vi "Is it a hex string.vi"(8 "error in (no error)":errorcluster, 9 "length (rest)":i32, 10 "String offset":u32, 11 "String to check":string) -> (0 "error out":errorcluster, 3 "Is Hex string?":bool)   [LabVIEW 2013]
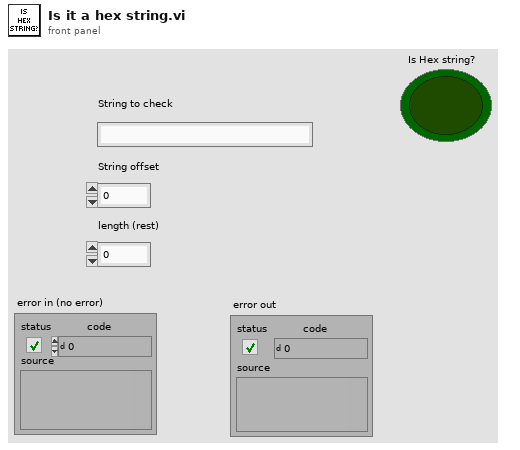
[diagram p1: front panel]
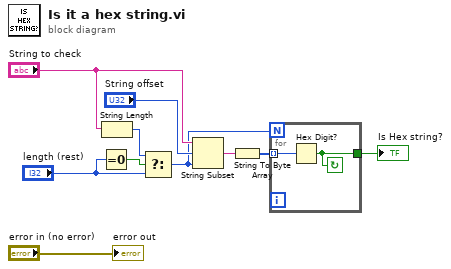
[diagram p0: block diagram]
diagram:
  n1 = Equal To 0?(x="length (rest)") -> (x = 0?=w5:bool)
  n2 = String Length(string="String to check") -> (length=w2:i32)
  n3 = Select(t=w2, s=w5, f="length (rest)") -> (s? t:f=w1:i32)
  n4 = String Subset(string="String to check", offset (0)="String offset", length (rest)=w1) -> (substring=w6:string)
  n5 = String To Byte Array(string=w6) -> (unsigned byte array=w10:u8[])
  n6 = for {
    N: w1 -> [_]
    tunnel: w10 -> [w12] mode=indexing
    tunnel: [w11] -> w9
    stop <- w11 continue-if-true
    n7 = Hex Digit?(1:w12) -> (0:w11:bool)
  }
  "Is Hex string?" <- w9
  "error out" <- "error in (no error)"
